vi "判读按下的是哪行，是否合法.vi"(8 "错误输入（无错误）":errorcluster, 9 "Coords":T1 caption="鼠标坐标", 11 "表格引用输入":refnum<vi>) -> (0 "错误输出":errorcluster, 1 "是否为合法行":bool, 2 "行输出":i32, 3 "表格引用输出":refnum<vi>)   [LabVIEW 2009]
uses:
  <vilib>/Utility/miscctls.llb/LVPoint32TypeDef.ctl
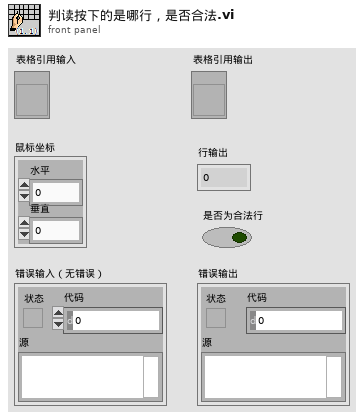
[diagram p1: front panel]
types:
  T1 = typedef "LVPoint32TypeDef.ctl" = cluster{"Horizontal":i32, "Vertical":i32}
  T2 = typedef "LVRowAndColumnTypeDef.ctl" = cluster{"Row":i32, "Column":i32}
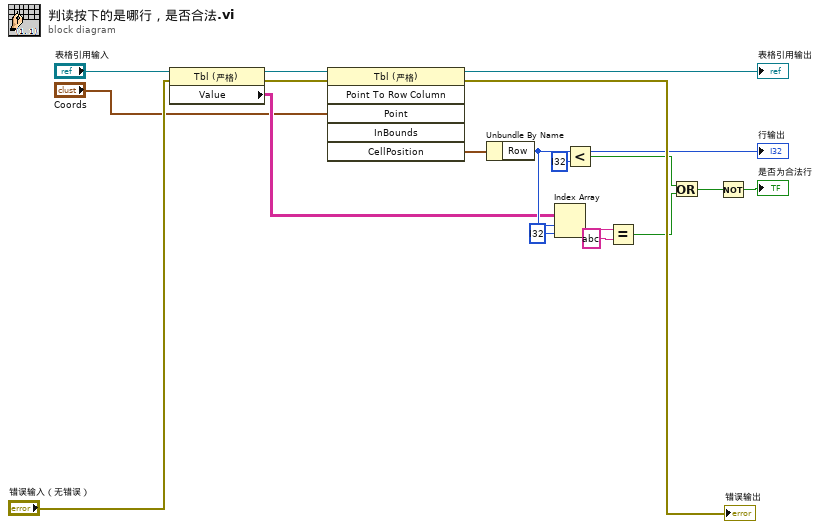
[diagram p0: block diagram]
diagram:
  n1 = property class="Tbl (严格)"(reference="表格引用输入", error in="错误输入（无错误）") -> (reference out=w3:refnum<vi>, error out=w16:errorcluster, "Value"=w8:string[][])
  n2 = invoke class="Tbl (严格)" method="Point To Row Column"(reference=w3, error in=w16, "Point"="Coords") -> (reference out=→"表格引用输出":refnum<vi>, error out=→"错误输出":errorcluster, "CellPosition"=w6:T2)  [unwired: 3 in, 3 out]
  n3 = Unbundle By Name(w6) -> ("Row"=w9:i32)
  "行输出" <- w9
  n4 = Index Array(array=w8, index (row)=w9, index (col)=i32 ? ("禁用的索引 (列)")) -> (element=w11:string)
  n5 = Less?(x=w9, y=i32 ?) -> (x < y?=w13:bool)
  n6 = Equal?(x=w11, y=string ?) -> (x = y?=w14:bool)
  n7 = Or(x=w13, y=w14) -> (x .or. y?=w15:bool)
  n8 = Not(x=w15) -> (.not. x?=→"是否为合法行":bool)
